vi "prg_out.vi"(6 "options":i32=128 format="%.0x", 7 "Reset to default":bool, 8 "error in (no error)":errorcluster, 9 "Name":string, 10 "machine name (\"\":  open local reference)":string, 11 "vi path":path) -> (0 "error out":errorcluster)   [LabVIEW 2015]
doc: "Set the reaction VI that will be called when a tuple with \"name\" in inserted in tuple space."
uses:
  C:/Users/Giuseppe/Downloads/LabLinda_ pakage/index_datatype.ctl
  C:/Users/Giuseppe/Downloads/LabLinda_ pakage/index_cluster.ctl
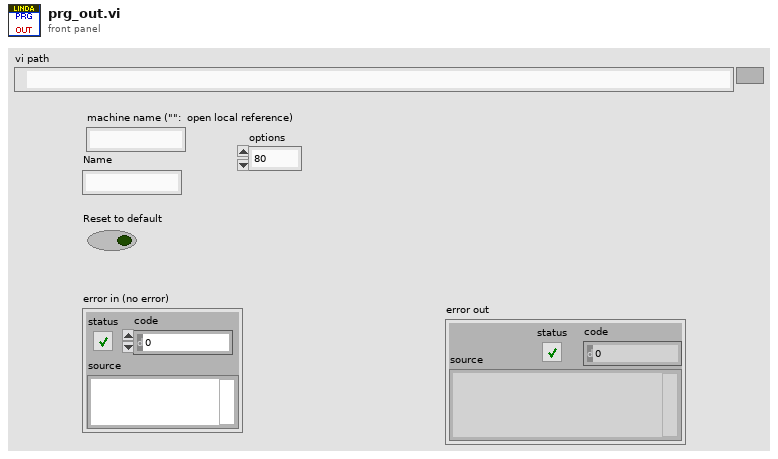
[diagram p1: front panel]
types:
  T1 = typedef "index_datatype.ctl" = T2[]
  T2 = typedef "index_cluster.ctl" = cluster{"Addr":i32[], "out react vi reference":refnum<vi>, "in react vi reference":refnum<vi>, "rd react vi reference":refnum<vi>, "Read_write_var":refnum<vi>}
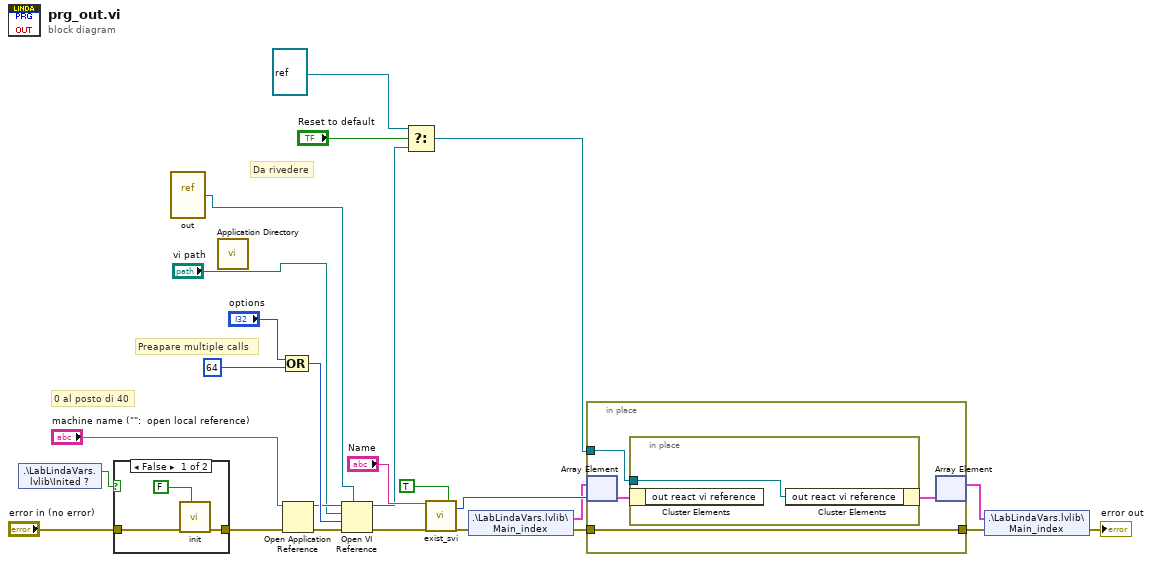
[diagram p0: block diagram]
diagram:
  # "Preapare multiple calls"
  # "Da rivedere"
  # "0 al posto di 40"
  n1 = shared-variable ".\\LabLindaVars.lvlib\\Inited ?"() -> (w6:bool)  [unwired: 1 in, 1 out]
  n2 = case shown="False" w6 {
    tunnel: [w28 w29] -> w4
    tunnel: "error in (no error)" -> [w27 w29]
    frame False {
      n3 = call "init.vi"("Cleaneup"=FALSE ("Cleneup"), "error in (no error)"=w27) -> ("error out"=w28:errorcluster)  [unwired: 9 in]
    }
    frame True {
    }
  }
  n4 = vi-ref "out.vi"() -> (w2:refnum<vi>)
  n5 = call <vilib>:"Application Directory.vi"() -> ()  [unwired: 1 out]
  n6 = Open Application Reference(8:w4, 11:"machine name (\"\":  open local reference)") -> (0:w10:errorcluster, 3:w8:refnum<vi>)  [unwired: 2 in]
  n7 = Compound Arithmetic op=OR("options", 64 ("Options")) -> (w23:i32)
  n8 = Open VI Reference(type specifier VI Refnum (for type only)=w2, application reference (local)=w8, vi path="vi path", options=w23, error in (no error)=w10) -> (vi reference=w17:refnum<vi>, error out=w7:errorcluster)  [unwired: 1 in]
  n9 = Select(t=refnum<vi> refnum, s="Reset to default", f=w17) -> (s? t:f=w16:refnum<vi>)
  n10 = call "exist_svi.vi"("Name"="Name", "error in (no error)"=w7, "Create ?"=TRUE) -> ("index of element"=w20:i32, "error out"=w14:errorcluster)  [unwired: 13 in, 2 out]
  n11 = shared-variable ".\\LabLindaVars.lvlib\\Main_index"(error in=w14) -> (w18:T1, error out=w13:errorcluster)
  n12 = in-place {
    in-place-border: w16 -> [w31]
    in-place-border: [w30] -> w12
    in-place-border: w13 -> [w30]
    n13 = in-place-array #1(w18, w20) -> (w33:T2)
    n14 = in-place {
      in-place-border: w31 -> [w34]
      n15 = in-place-cluster #2(w33) -> ()  [unwired: 1 out]
      n16 = in-place-cluster #2("out react vi reference"=w34) -> (w32:T2)
    }
    n17 = in-place-array #1(w32) -> (w19:T1)  [unwired: 1 out]
  }
  n18 = shared-variable ".\\LabLindaVars.lvlib\\Main_index"(w19, error in=w12) -> (error out=→"error out":errorcluster)
